vi "ExecuteBuildSpec.vi"(8 "error in (no error)":errorcluster, 10 "Spec Info":T1, 11 "ExecuteMultipleBuildSpecs in":refnum<class "ExecuteMultipleBuildSpecs.lvclass">) -> (0 "error out":errorcluster, 1 "Operation Output/Error Out":string, 2 "CLI Process Return Code":i32, 3 "ExecuteMultipleBuildSpecs out":refnum<class "ExecuteMultipleBuildSpecs.lvclass">)   [LabVIEW 2014, in "ExecuteMultipleBuildSpecs.lvclass"]
uses:
  ExecuteMultipleBuildSpecs.lvclass
  SpecInformation.ctl
  <nishared>/LabVIEW CLI/Operations/CoreOperation/CoreOperation.lvclass/CoreOperation.ctl
  ExecuteMultipleBuildSpecs.lvclass/ExecuteMultipleBuildSpecs.ctl
  <vilib>/AppBuilder/AB_API_Simple/Build (path).vi
  <nishared>/LabVIEW CLI/Operations/Utilities/Logger/Logger.lvclass
  <nishared>/LabVIEW CLI/Operations/CoreOperation/CoreOperation.lvclass
  <vilib>/AppBuilder/AB_API_Simple/NI_App_Builder_API.lvlib
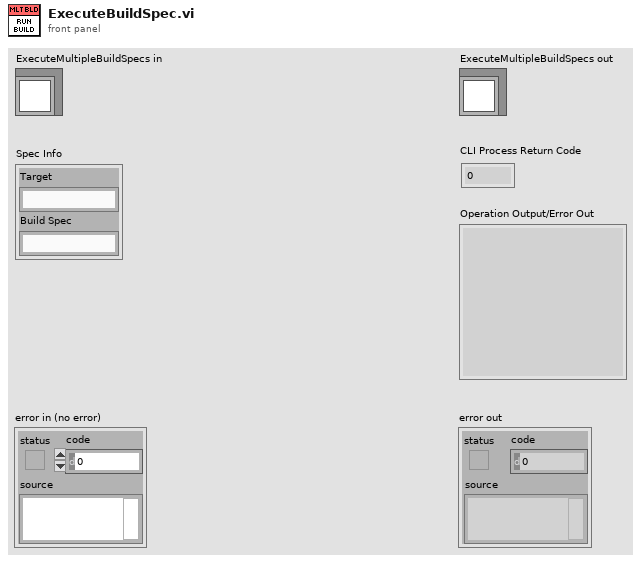
[diagram p1: front panel]
types:
  T1 = typedef "ExecuteMultipleBuildSpecs.lvclass/SpecInformation.ctl" = cluster{"Target":string, "Build Spec":string}
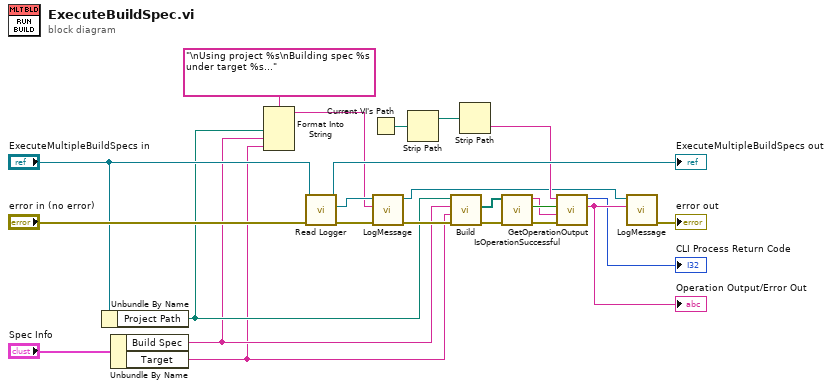
[diagram p0: block diagram]
diagram:
  n1 = Unbundle By Name("ExecuteMultipleBuildSpecs in") -> ("Project Path"=w13:path)
  n2 = Unbundle By Name("Spec Info") -> ("Build Spec"=w12:string, "Target"=w11:string)
  n3 = Format Into String(format string="\nUsing project %s\nBuilding spec %s under target %s...", w13, w12, w11) -> (resulting string=w17:string)  [unwired: 2 in, 1 out]
  n4 = call <nishared>:"Read Logger.vi"("error in (no error)"="error in (no error)", "CoreOperation in"="ExecuteMultipleBuildSpecs in") -> ("error out"=w23:errorcluster, "Logger.lvclass"=w21:refnum<class "Logger.lvclass">, "CoreOperation out"=→"ExecuteMultipleBuildSpecs out":refnum<class "ExecuteMultipleBuildSpecs.lvclass">)  [unwired: 7 in]
  n5 = Current VI's Path() -> (path=w9:path)
  n6 = call <nishared>:"LogMessage.vi"("error in (no error)"=w23, "Message"=w17, "Logger in"=w21) -> ("error out"=w16:errorcluster, "Logger out"=w5:refnum<class "Logger.lvclass">)  [unwired: 7 in]
  n7 = Strip Path(path=w9) -> (stripped path=w10:path)  [unwired: 1 out]
  n8 = call-poly <vilib>:"Build.vi"("error in (no error)"=w16, "Name of target (My Computer)"=w11, "Name of build specification (if empty: build all)"=w12, "Path to project"=w13) -> ("error out"=w15:errorcluster, "Generated files"=w14:path[])  [unwired: 6 in]
  n9 = Strip Path(path=w10) -> (name=w6:string)  [unwired: 1 out]
  n10 = call "IsOperationSuccessful.vi"("error in (no error)"=w15, "Generated files"=w14) -> ("error out"=w3:errorcluster, "Is Successful?"=w8:bool, "Output/Failure message"=w7:string)  [unwired: 7 in]
  n11 = call <nishared>:"GetOperationOutput.vi"("error in (no error)"=w3, "Operation Output/Error In"=w7, "Operation succeeded?"=w8, "Operation Name"=w6) -> ("Operation Output/Error Out"=w4:string, "CLI Process Return Code"=→"CLI Process Return Code":i32)  [unwired: 6 in]
  "Operation Output/Error Out" <- w4
  n12 = call <nishared>:"LogMessage.vi"("Message"=w4, "Logger in"=w5) -> ("error out"=→"error out":errorcluster)  [unwired: 8 in, 1 out]
